vi "ppb in ppm.vi"(10 "Werteingang":string) -> (3 "Wertausgang":string)   [LabVIEW 2020, in "Linearisierung v2.lvlib" / "Gasteiler.lvlib"]
uses:
  Gasteiler.lvlib
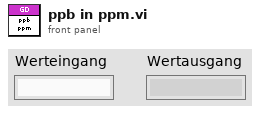
[diagram p1: front panel]
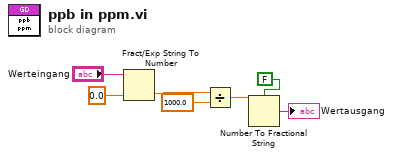
[diagram p0: block diagram]
diagram:
  n1 = Fract/Exp String To Number(string="Werteingang", default (0 dbl)=sgl 0.0 ("x")) -> (number=w6:sgl)  [unwired: 2 in, 1 out]
  n2 = Divide(x=w6, y=sgl 1000.0) -> (x/y=w1:sgl)
  n3 = Number To Fractional String(use system decimal point (T)=FALSE ("Systemdezimalzeichen verwenden (T)"), number=w1) -> (F-format string=→"Wertausgang":string)  [unwired: 2 in]
